vi "FPGA Types.vi"() -> ()   [LabVIEW 2021]
panel:
  in  "16_3":fxp<+,16,3>
  in  "18_3":fxp<+,18,3>
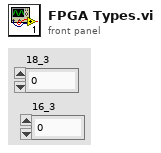
[diagram p1: front panel]
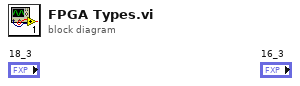
[diagram p0: block diagram]
diagram:
